vi "flattenToString.vi"(8 "error in (no error)":errorcluster, 11 "iMessage in":refnum<class "iMessage.lvclass">) -> (0 "error out":errorcluster, 3 "data string":string)   [LabVIEW 2017, in "Message Interface.lvlib" / "iMessage.lvclass"]
uses:
  iMessage.lvclass
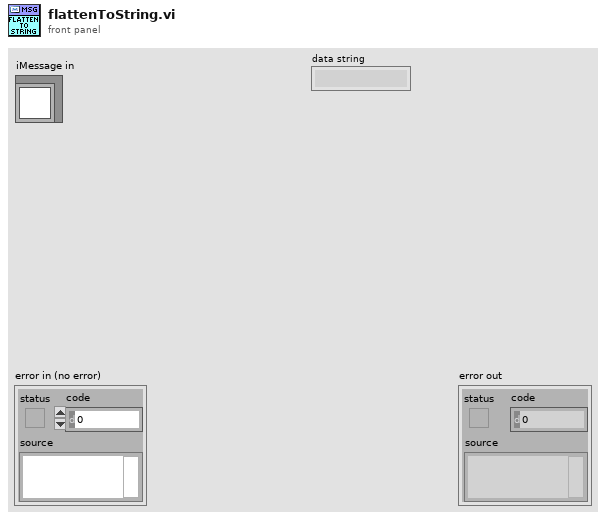
[diagram p1: front panel]
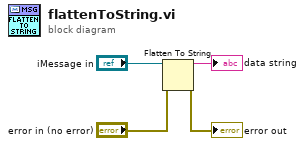
[diagram p0: block diagram]
diagram:
  n1 = Flatten To String(anything="iMessage in", error in (no error)="error in (no error)") -> (data string=→"data string":string, error out=→"error out":errorcluster)  [unwired: 2 in, 1 out]
